vi "SJ_Enter_Data_constant.vi"() -> (3 "SJ Data":T2={"Do (mm)"=3.0, "Dc (mm)"=0.039, "Ho (mm)"=0.01, "Hc (mm)"=0.006, "K"=1.251, "beta"=1.039, "Vc (m^3)"=0.0, "Vo (m^3)"=0.0})   [LabVIEW 2011]
uses:
  Controls/SJ_Data_Cluster.ctl
panel:
  in  "Cluster":T1={"Do (mm)"=5.0, "Dc (mm)"=40.0, "Ho (mm)"=5.0, "Hc (mm)"=4.0, "K"=1.251, "beta"=1.039}
  out "String":string
  in  "OK Button":bool
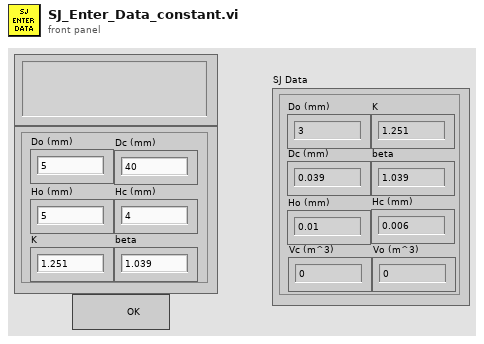
[diagram p1: front panel]
types:
  T1 = cluster{"Do (mm)":dbl, "Dc (mm)":dbl, "Ho (mm)":dbl, "Hc (mm)":dbl, "K":dbl, "beta":dbl}
  T2 = typedef "SJ_Data_Cluster.ctl" = cluster{"Do (mm)":dbl, "Dc (mm)":dbl, "Ho (mm)":dbl, "Hc (mm)":dbl, "K":dbl, "beta":dbl, "Vc (m^3)":dbl, "Vo (m^3)":dbl}
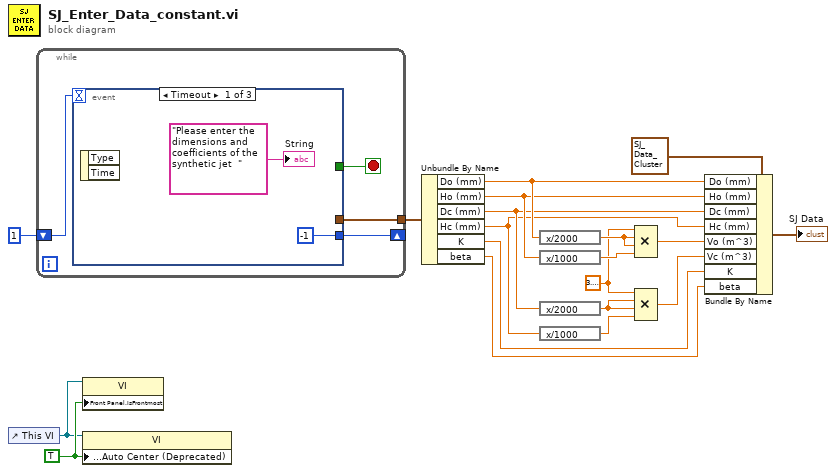
[diagram p0: block diagram]
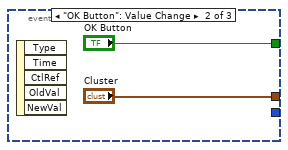
[diagram p2: hidden frame]
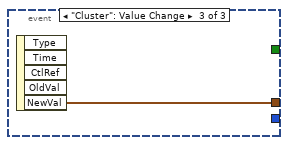
[diagram p3: hidden frame]
diagram:
  w13 = 3.141592653589793
  w18 = TRUE ("Front Panel Window:Is Frontmost")
  n1 = control-ref of="This VI"() -> (w17:refnum<vi>)
  n2 = while {
    shift-right: [w22] -> _
    shift-left: 1 -> [w23]
    tunnel: [w21] -> w7
    stop <- w20 stop-if-true
    n3 = event shown="[0] Timeout" {
      selector: _ -> [_ _ _]
      dyn-events: _ -> [_ _ _]
      timeout: w23 -> [_ _ _]
      tunnel: [-1 _ _] -> w22
      tunnel: [_ "Cluster" w28] -> w21
      tunnel: [_ "OK Button" _] -> w20
      event Timeout {
        n4 = event-data() -> ()  [unwired: 1 in, 2 out]
        "String" <- "Please enter the dimensions and coefficients of the synthetic jet  " ("String")
      }
      event "OK Button": Value Change {
        n5 = event-data() -> ()  [unwired: 1 in, 5 out]
      }
      event "Cluster": Value Change {
        n6 = event-data() -> ("NewVal"=w28:T1)  [unwired: 1 in, 4 out]
      }
    }
  }
  n7 = property class="VI"(reference=w17, "Front Panel.IsFrontmost"=w18) -> ()  [unwired: 1 in, 2 out]
  n8 = property class="VI"(reference=w17, "Front Panel Window:Auto Center (Deprecated)"=w18) -> ()  [unwired: 1 in, 2 out]
  n9 = Unbundle By Name(w7) -> ("Do (mm)"=w6:dbl, "Ho (mm)"=w5:dbl, "Dc (mm)"=w4:dbl, "Hc (mm)"=w3:dbl, "K"=w2:dbl, "beta"=w1:dbl)
  n10 = expression code="x/2000"(w6) -> (w15:dbl)
  n11 = expression code="x/1000"(w5) -> (w14:dbl)
  n12 = expression code="x/2000"(w4) -> (w12:dbl)
  n13 = expression code="x/1000"(w3) -> (w11:dbl)
  n14 = Compound Arithmetic op=MULTIPLY(w13, w15, w15, w14) -> (w10:dbl)
  n15 = Compound Arithmetic op=MULTIPLY(w13, w12, w12, w11) -> (w9:dbl)
  n16 = Bundle By Name(cluster=T2 {"Do (mm)"=3.0, "Dc (mm)"=0.039, "Ho (mm)"=0.01, "Hc (mm)"=0.006, "K"=1.251, "beta"=1.039, "Vc (m^3)"=0.0, "Vo (m^3)"=0.0} ("SJ Data IN"), "Do (mm)"=w6, "Ho (mm)"=w5, "Dc (mm)"=w4, "Hc (mm)"=w3, "Vo (m^3)"=w10, "Vc (m^3)"=w9, "K"=w2, "beta"=w1) -> (→"SJ Data":T2)
